vi "Setup_GlobalVariable.vi"   [LabVIEW 2018]
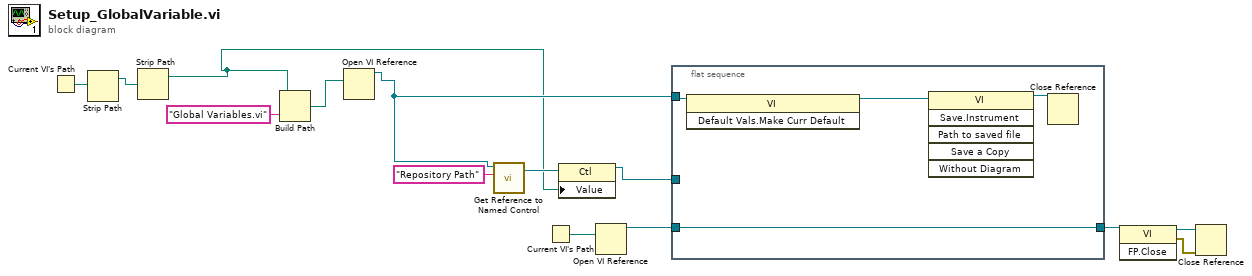
[diagram p0: block diagram]
diagram:
  n1 = Current VI's Path() -> (path=w14:path)
  n2 = Strip Path(path=w14) -> (stripped path=w2:path)  [unwired: 1 out]
  n3 = Strip Path(path=w2) -> (stripped path=w1:path)  [unwired: 1 out]
  n4 = Build Path(base path=w1, name or relative path="Global Variables.vi") -> (appended path=w12:path)
  n5 = Open VI Reference(vi path=w12) -> (vi reference=w8:refnum<vi>)  [unwired: 5 in, 1 out]
  n6 = call "Get Reference to Named Control.vi"("Control Name"="Repository Path", "Front Panel Ref"=w8) -> ("Ctl Refnum"=w10:refnum<vi>)  [unwired: 7 in, 2 out]
  n7 = Current VI's Path() -> (path=w7:path)
  n8 = property class="Ctl"(reference=w10, "Value"=w1) -> (reference out=w9:refnum<vi>)  [unwired: 1 in, 1 out]
  n9 = Open VI Reference(vi path=w7) -> (vi reference=w6:refnum<vi>)  [unwired: 5 in, 1 out]
  n10 = flat-sequence {
    tunnel: w9 -> [_]
    tunnel: w8 -> [w18]
    tunnel: [w16] -> w5
    tunnel: w6 -> [w16]
    frame #0 {
      n11 = invoke class="VI" method="Default Vals.Make Curr Default"(reference=w18) -> (reference out=w17:refnum<vi>)  [unwired: 2 in, 2 out]
      n12 = invoke class="VI" method="Save.Instrument"(reference=w17) -> (reference out=w15:refnum<vi>)  [unwired: 5 in, 5 out]
      n13 = Close Reference(reference=w15) -> ()  [unwired: 1 in, 1 out]
    }
  }
  n14 = invoke class="VI" method="FP.Close"(reference=w5) -> (reference out=w3:refnum<vi>, error out=w4:errorcluster)  [unwired: 2 in, 1 out]
  n15 = Close Reference(reference=w3, error in (no error)=w4) -> ()  [unwired: 1 out]
